vi "CollectFromMultipleNamespaces.vi"(10 "Requested Identifiers":string[](array[string]), 11 "Namespaces":variant[](array[variant])) -> (3 "RequiredNamespace":variant)   [LabVIEW 2019, in "Eval.lvlib"]
uses:
  Eval.lvlib
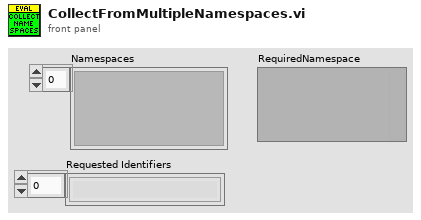
[diagram p1: front panel]
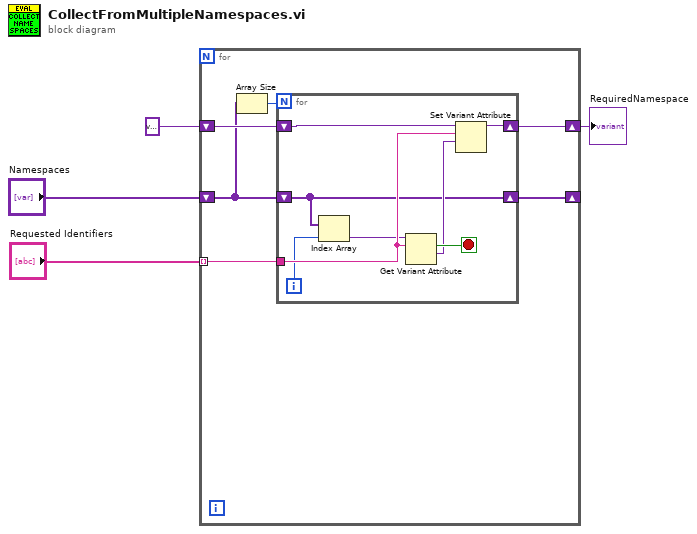
[diagram p0: block diagram]
diagram:
  n1 = for {
    tunnel: "Requested Identifiers" -> [w9] mode=indexing
    shift-right: [w8] -> w1
    shift-left: variant -> [w10]
    shift-right: [w7] -> _
    shift-left: "Namespaces" -> [w5]
    n2 = Array Size(array=w5) -> (size(s)=w6:i32)
    n3 = for {
      N: w6 -> [_]
      shift-right: [w17] -> w8
      shift-left: w10 -> [w16]
      tunnel: w9 -> [w14]
      shift-right: [w11] -> w7
      shift-left: w5 -> [w11]
      i -> [w13]
      stop <- w18 stop-if-true
      n4 = Index Array(array=w11, index=w13) -> (element=w12:variant)
      n5 = Get Variant Attribute(Variant=w12, name=w14) -> (found=w18:bool, value=w15:variant)  [unwired: 2 in, 2 out]
      n6 = Set Variant Attribute(Variant=w16, name=w14, value=w15) -> (Variant out=w17:variant)  [unwired: 1 in, 2 out]
    }
  }
  "RequiredNamespace" <- w1
